vi "9_Compensate_Input_Delays_setInputDelay.vi"() -> ()   [LabVIEW 2015]
uses:
  C:/Users/MX-Microscope/Documents/LabVIEW Data/lvoop_campus_2018/Detector_Class/Swabian/time_tagger_vis/TTCSharp32.dll
  TTCSharp32.dll
panel:
  in  "Clear Data":bool
  out "Counts per second":dbl[](array[numeric])
  in  "End Measurement":bool
  out "Counts per second with input Delay adjustment":dbl[](array[numeric])
  out "extracted delay [ps]\n (maximum of peak)":i64
  out "Cross correlation with input delay for compensation":cluster{"getIndex":i64[], "getData":i32[]}(graph)
  out "Cross correlation without inputDelay adjustment":cluster{"getIndex":i64[], "getData":i32[]}(graph)
  # "STAGE 1\nThe internal test signal has a propagation delay between the \ndifferent input channels.\nThis example shows how to use setInputDelay to compensate the offset."
  # "STAGE 2\nThe internal test signal of channel 1 is now shifted from the measurement\nof STAGE 1 so that clicks of both channels arrive at the very same time."
  # "chan 0"
  # "chan 0"
  # "chan 1"
  # "chan 1"
  # "coincidences"
  # "coincidences"
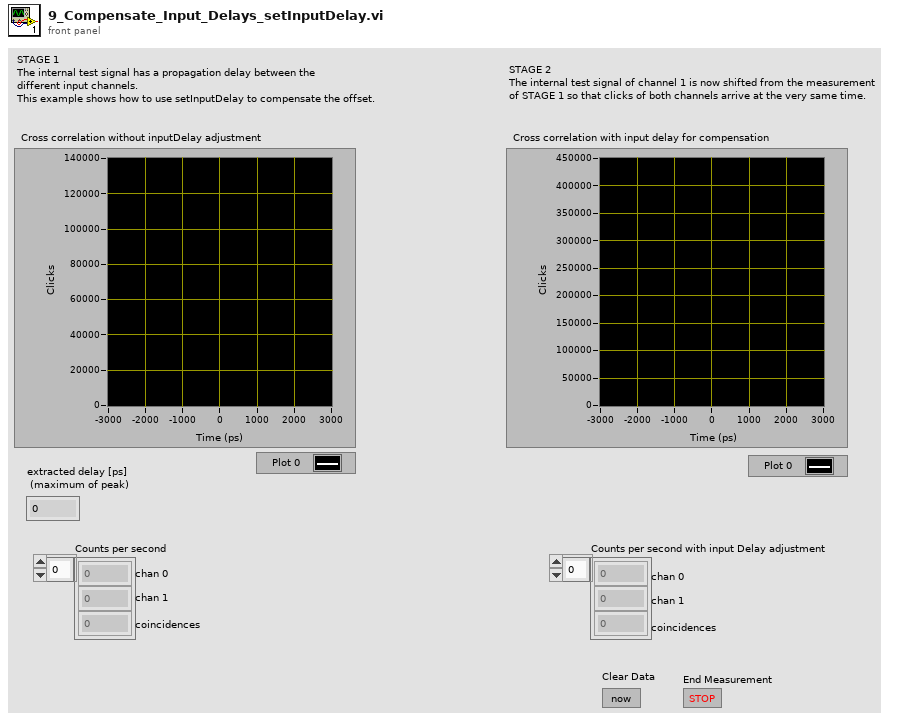
[diagram p1: front panel]
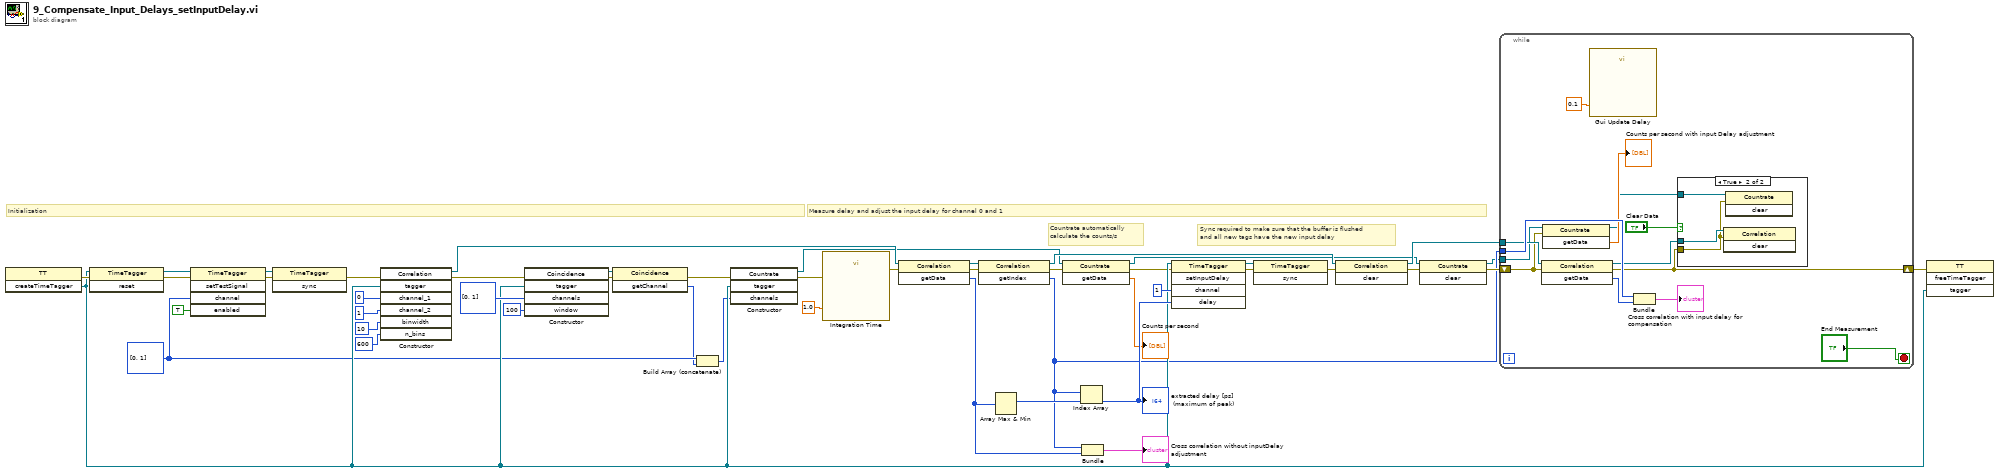
[diagram p0: block diagram]
diagram:
  w22 = u32[] [0, 1] ("channel")
  # "Countrate automatically \ncalculate the counts/s"
  # "Sync required to make sure that the buffer is flushed\nand all new tags have the new input delay"
  # "Measure delay and adjust the input delay for channel 0 and 1"
  # "Initialization"
  n1 = invoke class="TT" method="createTimeTagger"() -> (error out=w46:errorcluster, "createTimeTagger"=w23:refnum<k24>)  [unwired: 3 in, 1 out]
  n2 = invoke class="TimeTagger" method="reset"(reference=w23, error in=w46) -> (reference out=w40:refnum<k24>, error out=w41:errorcluster)  [unwired: 1 in, 1 out]
  n3 = invoke class="TimeTagger" method="setTestSignal"(reference=w40, error in=w41, "channel"=w22, "enabled"=TRUE) -> (reference out=w26:refnum<k24>, error out=w25:errorcluster)  [unwired: 1 in, 3 out]
  n4 = invoke class="TimeTagger" method="sync"(reference=w26, error in=w25) -> (error out=w24:errorcluster)  [unwired: 1 in, 2 out]
  n5 = constructor class="Correlation"(error in=w24, "tagger"=w23, "channel_1"=u32 0, "channel_2"=u32 1, "binwidth"=i64 10, "n_bins"=600) -> (reference out=w16:refnum<k24>, error out=w12:errorcluster)  [unwired: 2 in, 6 out]
  n6 = constructor class="Coincidence"(error in=w12, "tagger"=w23, "channels"=u32[] [0, 1], "window"=i64 100) -> (reference out=w4:refnum<k24>, error out=w2:errorcluster)  [unwired: 2 in, 4 out]
  n7 = invoke class="Coincidence" method="getChannel"(reference=w4, error in=w2) -> (error out=w1:errorcluster, "getChannel"=w3:u32)  [unwired: 1 in, 1 out]
  n8 = Build Array (concatenate)(w22, w3) -> (w21:u32[])
  n9 = constructor class="Countrate"(error in=w1, "tagger"=w23, "channels"=w21) -> (reference out=w9:refnum<k24>, error out=w11:errorcluster)  [unwired: 2 in, 3 out]
  n10 = call "Integration Time"("error in (no error)"=w11, "Delay Time (s)"=1.0) -> ("error out"=w38:errorcluster)  [unwired: 9 in]
  n11 = invoke class="Correlation" method="getData"(reference=w16, error in=w38) -> (reference out=w45:refnum<k24>, error out=w10:errorcluster, "getData"=w32:i32[])  [unwired: 1 in]
  n12 = invoke class="Correlation" method="getIndex"(reference=w45, error in=w10) -> (reference out=w17:refnum<k24>, error out=w6:errorcluster, "getIndex"=w18:i64[])  [unwired: 1 in]
  n13 = Array Max & Min(array=w32) -> (max index (indices)=w30:i32)  [unwired: 3 out]
  n14 = invoke class="Countrate" method="getData"(reference=w9, error in=w6) -> (reference out=w8:refnum<k24>, error out=w5:errorcluster, "getData"=→"Counts per second":dbl[])  [unwired: 1 in]
  n15 = Index Array(array=w18, index=w30) -> (element=w29:i64)
  "extracted delay [ps]\n (maximum of peak)" <- w29
  n16 = Bundle("getIndex"=w18, "getData"=w32) -> (→"Cross correlation without inputDelay adjustment":cluster{"getIndex":i64[], "getData":i32[]})  [unwired: 1 in]
  n17 = invoke class="TimeTagger" method="setInputDelay"(reference=w23, error in=w5, "channel"=u32 1, "delay"=w29) -> (reference out=w33:refnum<k24>, error out=w35:errorcluster)  [unwired: 1 in, 3 out]
  n18 = invoke class="TimeTagger" method="sync"(reference=w33, error in=w35) -> (error out=w34:errorcluster)  [unwired: 1 in, 2 out]
  n19 = invoke class="Correlation" method="clear"(reference=w17, error in=w34) -> (reference out=w15:refnum<k24>, error out=w20:errorcluster)  [unwired: 1 in, 1 out]
  n20 = invoke class="Countrate" method="clear"(reference=w8, error in=w20) -> (reference out=w14:refnum<k24>, error out=w19:errorcluster)  [unwired: 1 in, 1 out]
  n21 = while {
    tunnel: w18 -> [w58]
    tunnel: w15 -> [w56]
    tunnel: w14 -> [w55]
    shift-right: [w50] -> w13
    shift-left: w19 -> [w54]
    stop <- "End Measurement" stop-if-true
    n22 = invoke class="Correlation" method="getData"(reference=w56, error in=w54) -> (reference out=w52:refnum<k24>, error out=w50:errorcluster, "getData"=w59:i32[])  [unwired: 1 in]
    n23 = invoke class="Countrate" method="getData"(reference=w55, error in=w54) -> (reference out=w48:refnum<k24>, "getData"=→"Counts per second with input Delay adjustment":dbl[])  [unwired: 1 in, 1 out]
    n24 = call "Gui Update Delay"("Delay Time (s)"=0.1) -> ()  [unwired: 10 in, 1 out]
    n25 = Bundle("getIndex"=w58, "getData"=w59) -> (→"Cross correlation with input delay for compensation":cluster{"getIndex":i64[], "getData":i32[]})  [unwired: 1 in]
    n26 = case shown="True" "Clear Data" {
      tunnel: w52 -> [_ w63]
      tunnel: w50 -> [_ w62]
      tunnel: w48 -> [_ w61]
      frame False {
      }
      frame True {
        n27 = invoke class="Correlation" method="clear"(reference=w63, error in=w62) -> ()  [unwired: 1 in, 3 out]
        n28 = invoke class="Countrate" method="clear"(reference=w61, error in=w62) -> ()  [unwired: 1 in, 3 out]
      }
    }
  }
  n29 = invoke class="TT" method="freeTimeTagger"(error in=w13, "tagger"=w23) -> ()  [unwired: 2 in, 4 out]
